vi "Connect to Slave.vi"(8 "error in (no error)":errorcluster, 11 "stub in":refnum<class "stub.lvclass">) -> (0 "error out":errorcluster, 3 "stub out":refnum<class "stub.lvclass">)   [LabVIEW 2021, in "stub.lvclass"]
uses:
  stub.lvclass
  stub.lvclass/stub.ctl
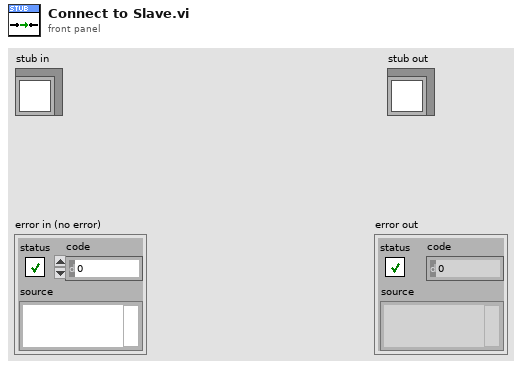
[diagram p1: front panel]
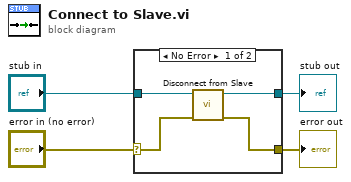
[diagram p0: block diagram]
diagram:
  n1 = case shown="No Error" "error in (no error)" {
    selector: "error in (no error)" -> [w7 w9]
    tunnel: [w5 w9] -> w3
    tunnel: [w6 w10] -> w1
    tunnel: "stub in" -> [w8 w10]
    frame No Error {
      n2 = call-dynamic "Disconnect from Slave.vi"("error in"=w7, "TCP master in"=w8) -> ("error out"=w5:errorcluster, "TCP master out"=w6:refnum<class "stub.lvclass">)  [unwired: 8 in]
    }
    frame Error {
    }
  }
  "error out" <- w3
  "stub out" <- w1
